vi "Z900_navX_Internal_ProcessingLoop.vi"(11 "navX Device":T1={"Interface"={"Protocol"=enum."SERIAL", "Update Rate (4Hz-100Hz)"=4, "navX Open TypeDef"=variant}, "Notify Packet"=refnum, "Loop VI Refnum"=refnum, "Ready to Close Occurrence Refnum"=refnum} {"Interface"."Update Rate (4Hz-100Hz)" min=4 max=60 step=1}) -> (0 "error out":errorcluster, 2 "Registry":u8[](array[numeric]))   [LabVIEW 2015, in "navX Library v2.lvlib"]
doc: "This navX VI handles the reading/writing for the navX. All of the good stuff is in here.\nTHIS VI SHOULD NOT BE CALLED BY THE USER!"
uses:
  navX Library v2.lvlib
  TypeDefs/Z900_navX_DeviceTypeDef.ctl
  TypeDefs/Z900_navX_ProtocolTypeDef.ctl
  TypeDefs/Z900_navX_NotifyPacketTypeDef.ctl
  TypeDefs/Z900_navX_ActionTypeDef.ctl
  <vilib>/Platform/TimedLoop/XDataNode/timing_clust.ctl
  <vilib>/Platform/TimedLoop/XDataNode/nitl_modes.ctl
  <vilib>/Platform/TimedLoop/XDataNode/wakeup.ctl
  TypeDefs/Z900_navX_InternalTimoutStatusTypeDef.ctl
  TypeDefs/navX Open TypeDefs/Z900_navX_OpenTypeDef_Serial.ctl
  NI WPI/WPI_SerialPort_USB.ctl
  TypeDefs/Z900_navX_SerialStreamTypeDef.ctl
  TypeDefs/Z900_navX_ZeroVectorTypeDef.ctl
  <vilib>/Rock Robotics/SystemInterfaces/Utilities/FPGA_UtilitiesRead LocalTime.vi
  <vilib>/Platform/TimedLoop/XDataNode/XDataNode.xnode
  <vilib>/Platform/TimedLoop/XDataNode/XDNodeRunTimeDep.lvlib
  NI WPI/NI WPI Serial USB.lvlib
panel:
  out "Connected":bool
  in  "Halt":bool
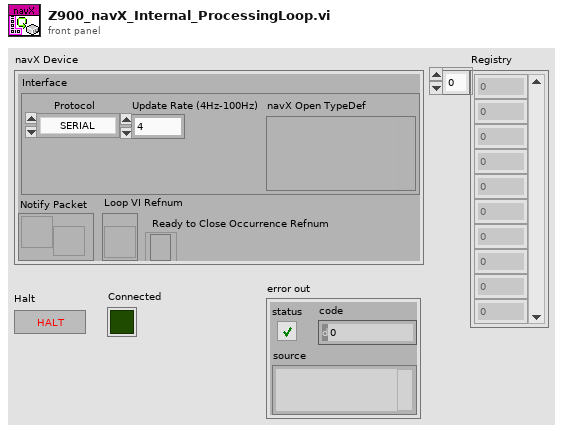
[diagram p1: front panel]
types:
  T1 = typedef "navX Library v2.lvlib/Z900_navX_DeviceTypeDef.ctl" = cluster{"Interface":cluster{"Protocol":T2, "Update Rate (4Hz-100Hz)":u8, "navX Open TypeDef":variant}, "Notify Packet":refnum<notifier>, "Loop VI Refnum":refnum<vi>, "Ready to Close Occurrence Refnum":refnum<k4>}
  T2 = typedef "navX Library v2.lvlib/Z900_navX_ProtocolTypeDef.ctl" = enum16{"SERIAL", "I2C", "SPI"}
  T3 = typedef "navX Library v2.lvlib/Z900_navX_InterfaceTypeDef.ctl" = cluster{"SerialPortRef":T4, "I2CDevRef":T5, "SPIDevRef":T7}
  T4 = typedef "WPI_SerialPortRef.ctl" = cluster{"DevStatus":errorcluster, "Serial Port Name":refnum<visa-resource-name>}
  T5 = typedef "WPI_I2CDevRef.ctl" = cluster{"DevStatus":errorcluster, "Device Address":u8, "Handle":i32, "I2C Bus":T6}
  T6 = typedef "i2c_bus.ctl" = enum16{"I2C On-Board", "I2C MXP", "Invalid"}
  T7 = typedef "WPI_SPIDevRef.ctl" = cluster{"DevStatus":errorcluster, "Handle":i32, "SPI Bus":T8}
  T8 = typedef "spi_bus.ctl" = enum16{"SPI On-Board, CS0", "SPI On-Board, CS1", "SPI On-Board, CS2", "SPI On-Board, CS3", "SPI MXP", "Invalid"}
  T9 = typedef "navX Library v2.lvlib/Z900_navX_InternalTimoutStatusTypeDef.ctl" = cluster{"Last Valid FPGA Time":dbl, "Error Count":i32, "Initialized":bool}
  T10 = typedef "XDNodeRunTimeDep.lvlib/timing_clust.ctl" = cluster{"Expected End [f-1]":u64, "Actual End [f-1]":u64, "Finished Late? [f-1]":bool, "Expected End [i-1]":u64, "Actual End [i-1]":u64, "Finished Late? [i-1]":bool, "Expected Start [i]":u64, "Actual Start [i]":u64, "Expected Start [f]":u64, "Actual Start [f]":u64, "Source Name":string, "Structure Name":string, "Period":i64, "Deadline":i64, "Offset":i64, "Start":i64, "Priority":i32, "Timeout":i32, "Mode":T11, "Wakeup Reason":T12, "Error":errorcluster, "Source Type":string, "Secondary Source Type":string, "Global End Time":u64, "Global Start Time":u64, "Frame Duration":u64, "Iteration Duration":u64, "Assigned CPU":i32, "I/O Scan Engine Mode":u32}
  T11 = typedef "XDNodeRunTimeDep.lvlib/nitl_modes.ctl" = enum32{"No Change", "Process missed periods, maintain original phase", "Discard missed periods, maintain original phase", "Process missed periods, ignore original phase", "Discard missed periods, ignore original phase"}
  T12 = typedef "XDNodeRunTimeDep.lvlib/wakeup.ctl" = enum32{"Normal", "Aborted", "Asynchronous wakeup", "Timing source error", "Timed loop error", "Timeout"}
  T13 = typedef "navX Library v2.lvlib/Z900_navX_OpenTypeDef_Serial.ctl" = cluster{"Serial Port":T14, "Stream Type":T15}
  T14 = typedef "NI WPI Serial USB.lvlib/WPI_SerialPort_USB.ctl" = enum16{"Onboard RS-232", "MXP TTL", "USB"}
  T15 = typedef "navX Library v2.lvlib/Z900_navX_SerialStreamTypeDef.ctl" = enum16{"YRPH", "Quaterinons", "Gyro/Raw", "AHRS", "AHRSAndPositioning"}
  T16 = typedef "navX Library v2.lvlib/Z900_navX_ZeroVectorTypeDef.ctl" = cluster{"X":bool, "Y":bool, "Z":bool}
  T17 = typedef "navX Library v2.lvlib/Z900_navX_NotifyPacketTypeDef.ctl" = cluster{"navX Action":T18, "Data":variant}
  T18 = typedef "navX Library v2.lvlib/Z900_navX_ActionTypeDef.ctl" = enum16{"None", "Halt", "Update Serial Protocol", "Zero-Yaw", "Zero-Displacement", "Zero-Velocity"}
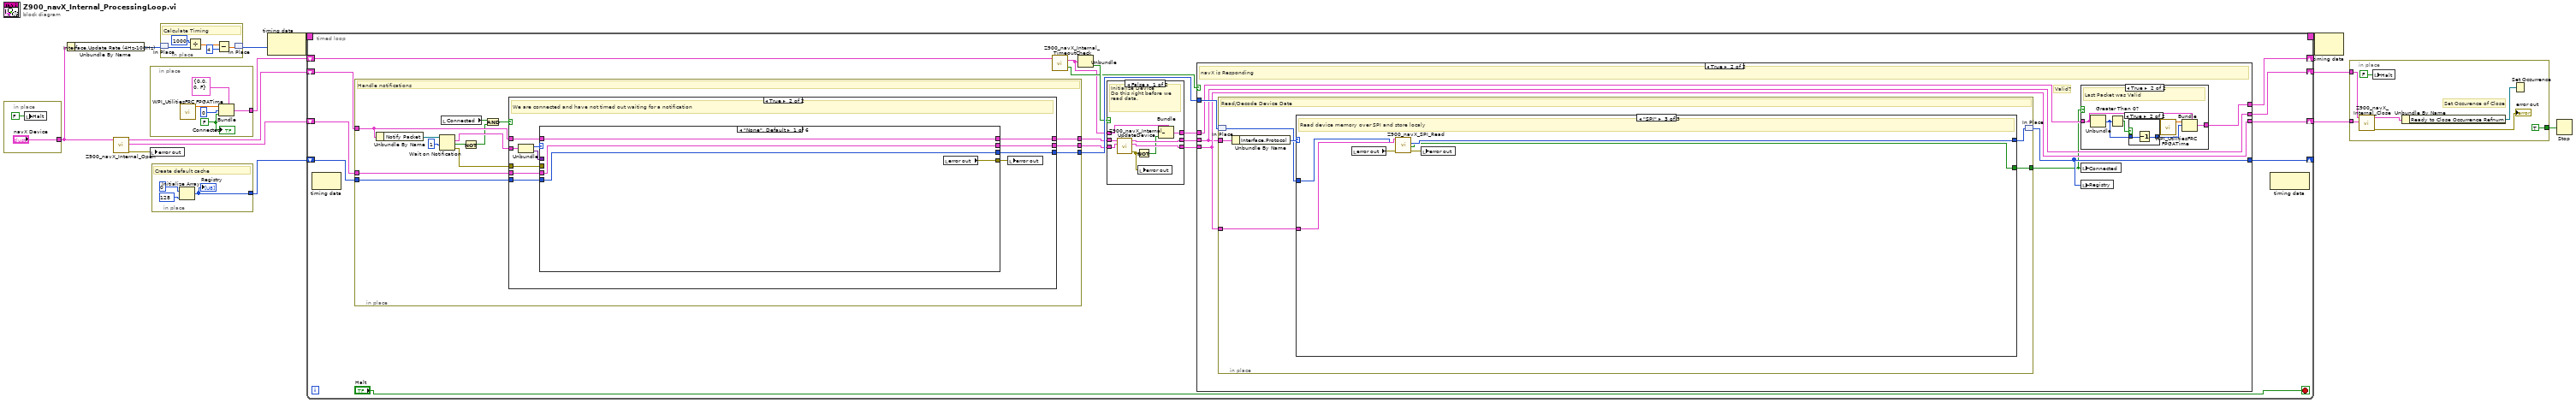
[diagram p0: block diagram]
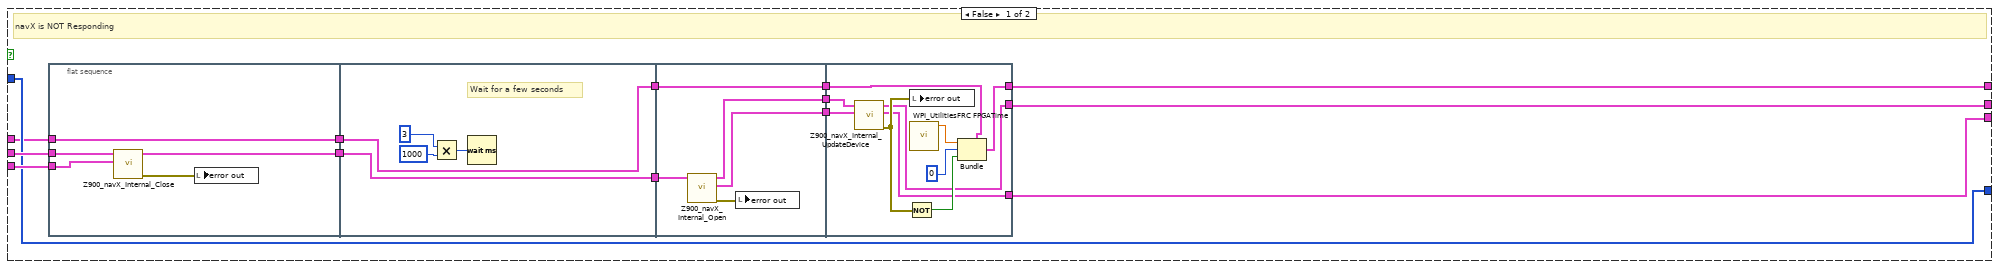
[diagram p3: hidden frame]
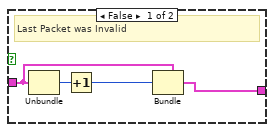
[diagram p4: hidden frame]
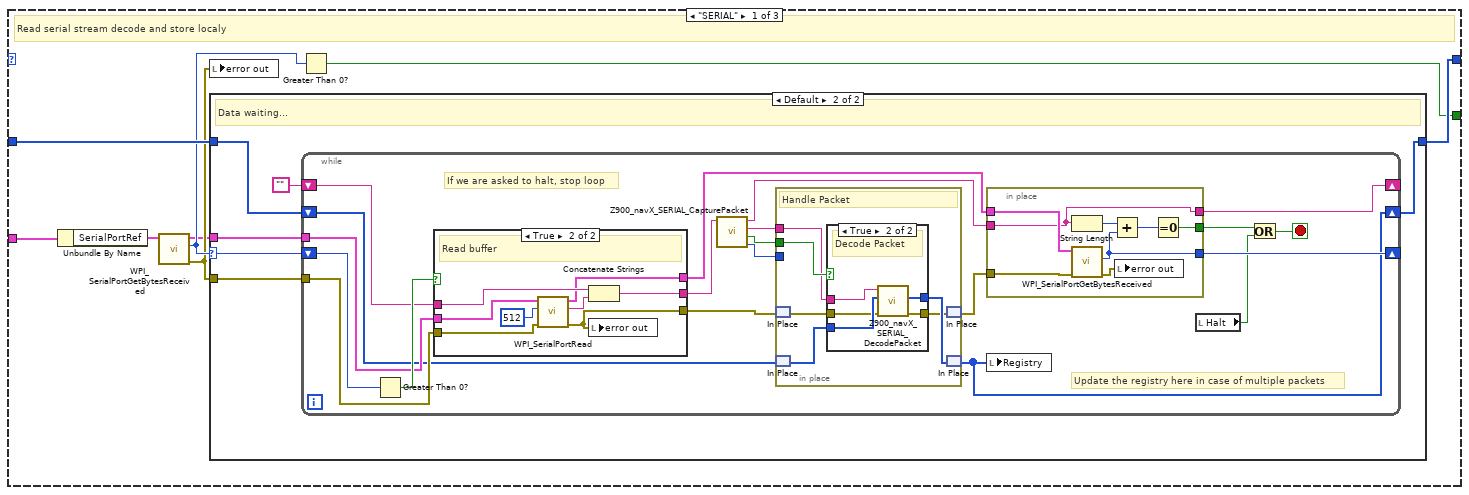
[diagram p6: hidden frame]
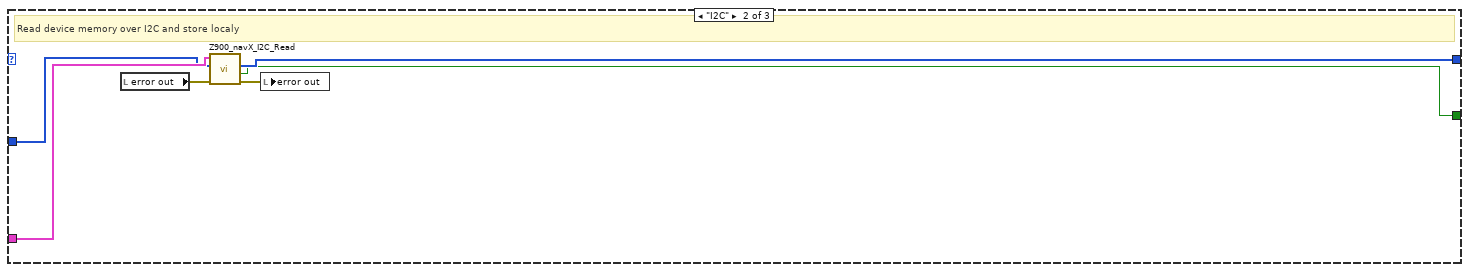
[diagram p10: hidden frame]
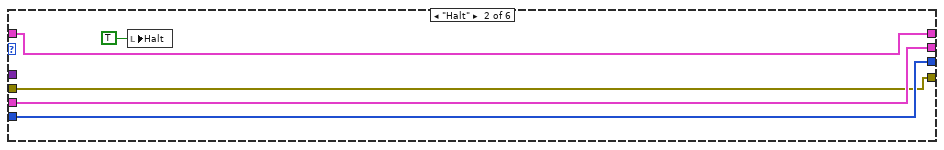
[diagram p12: hidden frame]
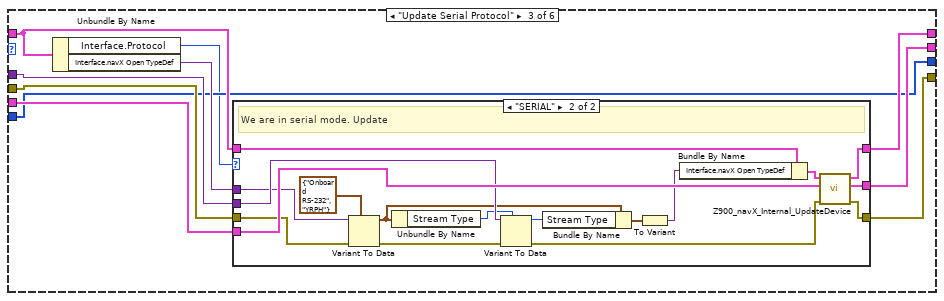
[diagram p13: hidden frame]
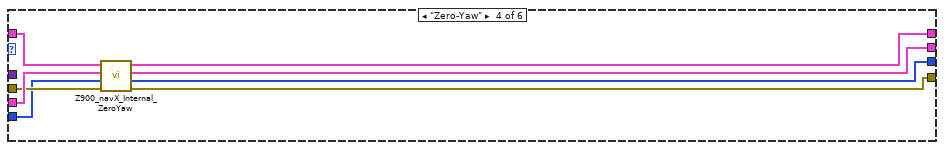
[diagram p15: hidden frame]
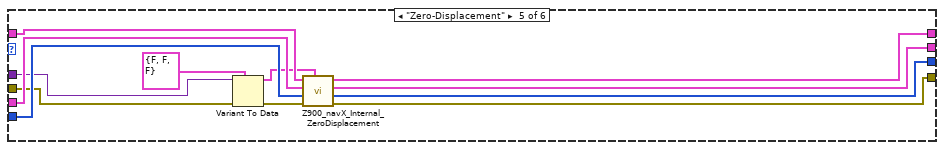
[diagram p16: hidden frame]
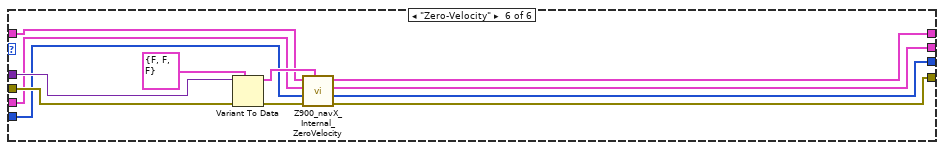
[diagram p17: hidden frame]
diagram:
  n1 = in-place {
    in-place-border: ["navX Device"] -> w6
    n2 = local write "Halt"(FALSE ("Halt")) -> ()
  }
  n3 = Unbundle By Name(w6) -> ("Interface.Update Rate (4Hz-100Hz)"=w10:u8)
  n4 = call "Z900_navX_Internal_Open.vi"("navX Device"=w6) -> ("error out"=w2:errorcluster, "Interface TypeDefs"=w5:T3, "navX Device"=w3:T1)  [unwired: 8 in]
  n5 = in-place {
    in-place-border: [w18] -> w4
    w16 = FALSE ("Initialized")
    n6 = call <vilib>:"WPI_UtilitiesFRC FPGATime.vi"() -> ("FPGA Time"=w19:dbl)  [unwired: 10 in, 1 out]
    n7 = Bundle(cluster=T9 {"Last Valid FPGA Time"=0.0, "Error Count"=0, "Initialized"=FALSE}, "Last Valid FPGA Time"=w19, "Error Count"=0, "Initialized"=w16) -> (w18:T9)
    "Connected" <- w16
  }
  n8 = local write "error out"(w2) -> ()
  n9 = in-place {
    in-place-border: [w21] -> w9
    # "Create default cache"
    n10 = Initialize Array(u8 0 ("Received Data"), 128 ("hex")) -> (w21:u8[])
    "Registry" <- w21
  }
  n11 = in-place {
    # "Calculate Timing"
    n12 = in-place-match #1(w10) -> (w27:u8)
    n13 = Divide(x=1000, y=w27) -> (x/y=w25:dbl)
    n14 = Subtract(x=w25, y=4) -> (x-y=w24:dbl)
    n15 = in-place-match #1(w24) -> (w11:u8)
  }
  n16 = node-c288(w11) -> (w13:T10)
  n17 = timed-loop {
    timing: w13 -> [_]
    timing-out: [_] -> w12
    shift-right: [w46] -> _
    shift-left: w9 -> [w42]
    shift-right: [w43] -> w8
    shift-left: w3 -> [w33]
    shift-right: [w44] -> w7
    shift-left: w5 -> [w32]
    shift-right: [w45] -> _
    shift-left: w4 -> [w31]
    stop <- "Halt" stop-if-true
    n18 = node-c288() -> ()  [unwired: 1 in, 1 out]
    n19 = in-place {
      in-place-border: w33 -> [w212]
      in-place-border: w32 -> [w211]
      in-place-border: [w210] -> w36
      in-place-border: [w209] -> w37
      in-place-border: w42 -> [w207]
      in-place-border: [w206] -> w41
      # "Handle notifications"
      n20 = Unbundle By Name(w212) -> ("Notify Packet"=w214:refnum<notifier>)
      n21 = Wait on Notification(notifier=w214, timeout in ms (-1)=1) -> (notification=w215:T17, timed out?=w205:bool, error out=w208:errorcluster)  [unwired: 2 in, 1 out]
      n22 = local read "Connected"() -> (w203:bool)
      n23 = Not(x=w205) -> (.not. x?=w204:bool)
      n24 = And(x=w203, y=w204) -> (x .and. y?=w202:bool)
      n25 = case shown="True" w202 {
        tunnel: w215 -> [_ w229]
        tunnel: w212 -> [w218 w227]
        tunnel: w211 -> [w217 w226]
        tunnel: [w217 w225] -> w210
        tunnel: [w218 w224] -> w209
        tunnel: w208 -> [_ w222]
        tunnel: w207 -> [w216 w221]
        tunnel: [w216 w220] -> w206
        frame False {
          # "We are either not connected or have timed out waiting for a notification"
        }
        frame True {
          # "We are connected and have not timed out waiting for a notification"
          n26 = Unbundle(w229) -> ("navX Action"=w228:T18, "Data"=w223:variant)
          n27 = case shown="\"None\", Default" w228 {
            tunnel: w227 -> [w233 w238 w242 w276 w288 w295]
            tunnel: w226 -> [w232 w237 w248 w274 w286 w294]
            tunnel: [w232 w237 w247 w273 w284 w291] -> w225
            tunnel: [w233 w238 w246 w275 w285 w292] -> w224
            tunnel: w223 -> [_ _ w245 _ w281 w298]
            tunnel: w222 -> [_ w235 w243 w272 w278 w299]
            tunnel: w221 -> [w231 w236 w241 w271 w287 w293]
            tunnel: [w231 w236 w241 w270 w283 w290] -> w220
            tunnel: [w230 w235 w240 w269 w282 w289] -> w219
            frame "None", Default {
              n28 = local read "error out"() -> (w230:errorcluster)
            }
            frame "Halt" {
              n29 = local write "Halt"(TRUE) -> ()
            }
            frame "Update Serial Protocol" {
              n30 = Unbundle By Name(w242) -> ("Interface.Protocol"=w239:T2, "Interface.navX Open TypeDef"=w244:variant)
              n31 = case shown="\"SERIAL\"" w239 {
                tunnel: w248 -> [w250 w268]
                tunnel: [w250 w267] -> w247
                tunnel: [w251 w266] -> w246
                tunnel: w245 -> [_ w265]
                tunnel: w244 -> [_ w262]
                tunnel: w243 -> [w249 w259]
                tunnel: w242 -> [w251 w258]
                tunnel: [w249 w252] -> w240
                frame Default {
                  # "We don't care if we are not in serial mode."
                }
                frame "SERIAL" {
                  # "We are in serial mode. Update"
                  n32 = Variant To Data(error in=w259, type=T13 {"Serial Port"=enum."Onboard RS-232", "Stream Type"=enum."YRPH"} ("navX Serial Open"), Variant=w262) -> (data=w255:T13, error out=w260:errorcluster)
                  n33 = Unbundle By Name(w255) -> ("Stream Type"=w254:T15)
                  n34 = Variant To Data(error in=w260, type=w254, Variant=w265) -> (data=w253:T15, error out=w264:errorcluster)
                  n35 = Bundle By Name(cluster=w255, "Stream Type"=w253) -> (w263:T13)
                  n36 = To Variant(anything=w263) -> (Variant=w257:variant)
                  n37 = Bundle By Name(cluster=w258, "Interface.navX Open TypeDef"=w257) -> (w256:T1)
                  n38 = call "Z900_navX_Internal_UpdateDevice.vi"("error in (no error)"=w264, "Interface TypeDefs"=w268, "navX Device"=w256) -> ("error out"=w252:errorcluster, "Interface TypeDefs"=w267:T3, "navX Device"=w266:T1)  [unwired: 6 in]
                }
              }
            }
            frame "Zero-Yaw" {
              n39 = call "Z900_navX_Internal_ZeroYaw.vi"("error in (no error)"=w272, "Registry"=w271, "Interface TypeDefs"=w274, "navX Device"=w276) -> ("error out"=w269:errorcluster, "Registry"=w270:u8[], "Interface TypeDefs"=w273:T3, "navX Device"=w275:T1)  [unwired: 4 in]
            }
            frame "Zero-Displacement" {
              n40 = Variant To Data(error in=w278, type=T16 {"X"=FALSE, "Y"=FALSE, "Z"=FALSE} ("Zero Vector"), Variant=w281) -> (data=w279:T16, error out=w277:errorcluster)
              n41 = call "Z900_navX_Internal_ZeroDisplacement.vi"("Zero Vector"=w279, "error in (no error)"=w277, "Registry"=w287, "Interface TypeDefs"=w286, "navX Device"=w288) -> ("error out"=w282:errorcluster, "Registry"=w283:u8[], "Interface TypeDefs"=w284:T3, "navX Device"=w285:T1)  [unwired: 3 in]
            }
            frame "Zero-Velocity" {
              n42 = Variant To Data(error in=w299, type=T16 {"X"=FALSE, "Y"=FALSE, "Z"=FALSE} ("Zero Vector"), Variant=w298) -> (data=w297:T16, error out=w296:errorcluster)
              n43 = call "Z900_navX_Internal_ZeroVelocity.vi"("Zero Vector"=w297, "error in (no error)"=w296, "Registry"=w293, "Interface TypeDefs"=w294, "navX Device"=w295) -> ("error out"=w289:errorcluster, "Registry"=w290:u8[], "Interface TypeDefs"=w291:T3, "navX Device"=w292:T1)  [unwired: 3 in]
            }
          }
          n44 = local write "error out"(w219) -> ()
        }
      }
    }
    n45 = call "Z900_navX_Internal_TimeoutCheck.vi"("Timout Status (in)"=w31) -> ("TIMEOUT!"=w30:bool, "Timout Status (out)"=w29:T9)  [unwired: 2 in]
    n46 = Unbundle(w29) -> ("Initialized"=w39:bool)  [unwired: 2 out]
    n47 = case shown="False" w39 {
      tunnel: w29 -> [w54 w57]
      tunnel: [w53 w57] -> w38
      tunnel: w37 -> [w52 w56]
      tunnel: w36 -> [w51 w55]
      tunnel: [w50 w56] -> w34
      tunnel: [w49 w55] -> w35
      frame False {
        # "Initialize Device\nDo this right before we\nread data."
        n48 = call "Z900_navX_Internal_UpdateDevice.vi"("Interface TypeDefs"=w51, "navX Device"=w52) -> ("error out"=w48:errorcluster, "Interface TypeDefs"=w49:T3, "navX Device"=w50:T1)  [unwired: 7 in]
        n49 = Not(x=w48) -> (.not. x?=w47:bool)
        n50 = local write "error out"(w48) -> ()
        n51 = Bundle(cluster=w54, "Initialized"=w47) -> (w53:T9)  [unwired: 2 in]
      }
      frame True {
      }
    }
    n52 = case shown="True" w30 {
      tunnel: w41 -> [w69 w103]
      tunnel: w35 -> [w70 w102]
      tunnel: [w69 w99] -> w46
      tunnel: w38 -> [w58 w101]
      tunnel: [w62 w100] -> w45
      tunnel: w34 -> [w71 w98]
      tunnel: [w63 w98] -> w43
      tunnel: [w66 w102] -> w44
      frame False {
        # "navX is NOT Responding"
        n53 = flat-sequence {
          tunnel: w71 -> [w74]
          tunnel: w70 -> [w76]
          tunnel: [w75] -> w68
          tunnel: [w72] -> w59
          tunnel: w58 -> [w72]
          tunnel: w68 -> [w81]
          tunnel: [w81] -> w67
          tunnel: [w77] -> w60
          tunnel: w59 -> [w77]
          tunnel: w67 -> [w85]
          tunnel: [w86] -> w65
          tunnel: [w84] -> w64
          tunnel: [w82] -> w61
          tunnel: w60 -> [w82]
          tunnel: [w94] -> w62
          tunnel: [w90] -> w66
          tunnel: [w91] -> w63
          tunnel: w61 -> [w89]
          tunnel: w64 -> [w92]
          tunnel: w65 -> [w93]
          frame #0 {
            n54 = call "Z900_navX_Internal_Close.vi"("Interface TypeDefs"=w76, "navX Device"=w74) -> ("error out"=w73:errorcluster, "navX Device"=w75:T1)  [unwired: 8 in]
            n55 = local write "error out"(w73) -> ()
          }
          frame #1 {
            # "Wait for a few seconds"
            n56 = Multiply(x=u32 3 ("milliseconds to wait"), y=u32 1000) -> (x*y=w79:u32)
            n57 = Wait (ms)(milliseconds to wait=w79) -> ()  [unwired: 1 out]
          }
          frame #2 {
            n58 = call "Z900_navX_Internal_Open.vi"("navX Device"=w85) -> ("error out"=w83:errorcluster, "Interface TypeDefs"=w84:T3, "navX Device"=w86:T1)  [unwired: 8 in]
            n59 = local write "error out"(w83) -> ()
          }
          frame #3 {
            n60 = call "Z900_navX_Internal_UpdateDevice.vi"("Interface TypeDefs"=w92, "navX Device"=w93) -> ("error out"=w95:errorcluster, "Interface TypeDefs"=w90:T3, "navX Device"=w91:T1)  [unwired: 7 in]
            n61 = Not(x=w95) -> (.not. x?=w96:bool)
            n62 = local write "error out"(w95) -> ()
            n63 = call <vilib>:"WPI_UtilitiesFRC FPGATime.vi"() -> ("FPGA Time"=w88:dbl)  [unwired: 10 in, 1 out]
            n64 = Bundle(cluster=w89, "Last Valid FPGA Time"=w88, "Error Count"=0, "Initialized"=w96) -> (w94:T9)
          }
        }
      }
      frame True {
        # "Valid?"
        # "navX is Responding"
        n65 = in-place {
          in-place-border: w98 -> [w117]
          in-place-border: w102 -> [w121]
          in-place-border: [w119] -> w97
          # "Read/Decode Device Date"
          n66 = in-place-match #2(w103) -> (w120:u8[])
          n67 = Unbundle By Name(w117) -> ("Interface.Protocol"=w122:T2)
          n68 = case shown="\"SPI\"" w122 {
            tunnel: [w128 w191 w197] -> w118
            tunnel: w120 -> [w129 w192 w200]
            tunnel: w121 -> [w130 w195 w201]
            tunnel: [w126 w190 w196] -> w119
            frame "SERIAL" {
              # "Read serial stream decode and store localy"
              n69 = Unbundle By Name(w130) -> ("SerialPortRef"=w127:T4)
              n70 = call <vilib>:"WPI_SerialPortGetBytesReceived.vi"("SerialPortRef"=w127) -> ("error out"=w124:errorcluster, "Bytes at Port"=w125:u32, "SerialPortRef"=w123:T4)  [unwired: 8 in]
              n71 = local write "error out"(w124) -> ()
              n72 = case shown="Default" w125 {
                selector: w125 -> [_ w132]
                tunnel: [w131 w137] -> w128
                tunnel: w129 -> [w131 w136]
                tunnel: w123 -> [_ w134]
                tunnel: w124 -> [_ w133]
                frame 0 {
                }
                frame Default {
                  # "Data waiting..."
                  n73 = while {
                    shift-right: [w139] -> w137
                    shift-left: w136 -> [w146]
                    shift-right: [w150] -> _
                    shift-left: w132 -> [w157]
                    shift-right: [w149] -> _
                    shift-left: "" -> [w155]
                    tunnel: w134 -> [w154]
                    tunnel: w133 -> [w153]
                    stop <- w142 stop-if-true
                    # "Update the registry here in case of multiple packets"
                    # "If we are asked to halt, stop loop"
                    n74 = Greater Than 0?(x=w157) -> (x > 0?=w156:bool)
                    n75 = case shown="True" w156 {
                      tunnel: w155 -> [w181 w189]
                      tunnel: w154 -> [w180 w188]
                      tunnel: w153 -> [w179 w185]
                      tunnel: [w181 w184] -> w152
                      tunnel: [w180 w183] -> w138
                      tunnel: [w179 w182] -> w145
                      frame False {
                        # "Pass existing buffer"
                      }
                      frame True {
                        # "Read buffer"
                        n76 = call <vilib>:"WPI_SerialPortRead.vi"("error in (no error)"=w185, "Num Bytes to Read"=u32 512, "SerialPortRef"=w188) -> ("error out"=w182:errorcluster, "Buffer"=w187:string, "SerialPortRef"=w183:T4)  [unwired: 6 in]
                        n77 = Concatenate Strings(w189, w187) -> (w184:string)
                        n78 = local write "error out"(w182) -> ()
                      }
                    }
                    n79 = call "Z900_navX_SERIAL_CapturePacket.vi"("Buffer"=w152) -> ("Packet Size"=w147:i32, "Packet Located"=w140:bool, "Packet"=w148:string, "Buffer"=w151:string)  [unwired: 7 in]
                    n80 = in-place {
                      in-place-border: w148 -> [w162]
                      in-place-border: w140 -> [w163]
                      in-place-border: w147 -> [_]
                      # "Handle Packet"
                      n81 = in-place-match #3(w145) -> (w159:errorcluster)
                      n82 = in-place-match #4(w146) -> (w160:u8[])
                      n83 = case shown="True" w163 {
                        tunnel: w162 -> [_ w170]
                        tunnel: [w165 w168] -> w161
                        tunnel: w160 -> [w165 w169]
                        tunnel: w159 -> [w164 w167]
                        tunnel: [w164 w166] -> w158
                        frame False {
                          # "No Packet"
                        }
                        frame True {
                          # "Decode Packet"
                          n84 = call "Z900_navX_SERIAL_DecodePacket.vi"("error in (no error)"=w167, "Data"=w169, "Packet"=w170) -> ("error out"=w166:errorcluster, "Data"=w168:u8[])  [unwired: 6 in, 1 out]
                        }
                      }
                      n85 = in-place-match #3(w158) -> (w144:errorcluster)
                      n86 = in-place-match #4(w161) -> (w139:u8[])
                    }
                    n87 = in-place {
                      in-place-border: w138 -> [w178]
                      in-place-border: w144 -> [w177]
                      in-place-border: w151 -> [w172]
                      in-place-border: [w174] -> w143
                      in-place-border: [w173] -> w150
                      in-place-border: [w172] -> w149
                      n88 = String Length(string=w172) -> (length=w175:i32)
                      n89 = call <vilib>:"WPI_SerialPortGetBytesReceived.vi"("error in (no error)"=w177, "SerialPortRef"=w178) -> ("error out"=w171:errorcluster, "Bytes at Port"=w173:u32)  [unwired: 7 in, 1 out]
                      n90 = Add(x=w175, y=w173) -> (x+y=w176:u32)
                      n91 = local write "error out"(w171) -> ()
                      n92 = Equal To 0?(x=w176) -> (x = 0?=w174:bool)
                    }
                    n93 = local write "Registry"(w139) -> ()
                    n94 = local read "Halt"() -> (w141:bool)
                    n95 = Or(x=w143, y=w141) -> (x .or. y?=w142:bool)
                  }
                }
              }
              n96 = Greater Than 0?(x=w125) -> (x > 0?=w126:bool)
            }
            frame "I2C" {
              # "Read device memory over I2C and store localy"
              n97 = local read "error out"() -> (w194:errorcluster)
              n98 = call "Z900_navX_I2C_Read.vi"("error in (no error)"=w194, "Registry"=w192, "Interface TypeDefs"=w195) -> ("error out"=w193:errorcluster, "Valid"=w190:bool, "Registry"=w191:u8[])  [unwired: 5 in, 1 out]
              n99 = local write "error out"(w193) -> ()
            }
            frame "SPI" {
              # "Read device memory over SPI and store localy"
              n100 = local read "error out"() -> (w199:errorcluster)
              n101 = call "Z900_navX_SPI_Read.vi"("error in (no error)"=w199, "Registry"=w200, "Interface TypeDefs"=w201) -> ("error out"=w198:errorcluster, "Valid"=w196:bool, "Registry"=w197:u8[])  [unwired: 5 in, 1 out]
              n102 = local write "error out"(w198) -> ()
            }
          }
          n103 = in-place-match #2(w118) -> (w99:u8[])
        }
        n104 = case shown="True" w97 {
          tunnel: [w104 w112] -> w100
          tunnel: w101 -> [w105 w111]
          frame False {
            # "Last Packet was Invalid"
            n105 = Unbundle(w105) -> ("Error Count"=w106:i32)  [unwired: 2 out]
            n106 = Increment(x=w106) -> (x+1=w107:i32)
            n107 = Bundle(cluster=w105, "Error Count"=w107) -> (w104:T9)  [unwired: 2 in]
          }
          frame True {
            # "Last Packet was Valid"
            n108 = Unbundle(w111) -> ("Error Count"=w109:i32)  [unwired: 2 out]
            n109 = Greater Than 0?(x=w109) -> (x > 0?=w110:bool)
            n110 = case shown="True" w110 {
              tunnel: [w114 w115] -> w108
              tunnel: w109 -> [w114 w116]
              frame False {
              }
              frame True {
                n111 = Decrement(x=w116) -> (x-1=w115:i32)
              }
            }
            n112 = call <vilib>:"WPI_UtilitiesFRC FPGATime.vi"() -> ("FPGA Time"=w113:dbl)  [unwired: 10 in, 1 out]
            n113 = Bundle(cluster=w111, "Last Valid FPGA Time"=w113, "Error Count"=w108) -> (w112:T9)  [unwired: 1 in]
          }
        }
        n114 = local write "Connected"(w97) -> ()
        n115 = local write "Registry"(w99) -> ()
      }
    }
    n116 = node-c288() -> ()  [unwired: 1 in, 1 out]
  }
  n117 = node-c288(w12) -> ()  [unwired: 1 out]
  n118 = in-place {
    in-place-border: w8 -> [w309]
    in-place-border: w7 -> [w308]
    in-place-border: [TRUE] -> w1
    # "Set Occurence of Close"
    n119 = call "Z900_navX_Internal_Close.vi"("Interface TypeDefs"=w308, "navX Device"=w309) -> ("error out"=→"error out":errorcluster, "navX Device"=w303:T1)  [unwired: 8 in]
    n120 = local write "Halt"(FALSE ("Halt")) -> ()
    n121 = Unbundle By Name(w303) -> ("Ready to Close Occurrence Refnum"=w305:refnum<k4>)
    n122 = Set Occurrence(w305) -> ()
  }
  n123 = Stop(stop? (T)=w1) -> ()
